vi "Device Params From Config XML File.vi"(8 "error IN":errorcluster, 11 "Configuration in":refnum<class "Configuration.lvclass">) -> (0 "error OUT":errorcluster, 1 "Device Settings":T2, 2 "Device Connections":T1, 3 "Configuration out":refnum<class "Configuration.lvclass">)   [LabVIEW 2011]
uses:
  Controls/Device Settings.ctl
  Controls/Device Connections.ctl
  Modules/File/Configuration/Configuration.lvclass
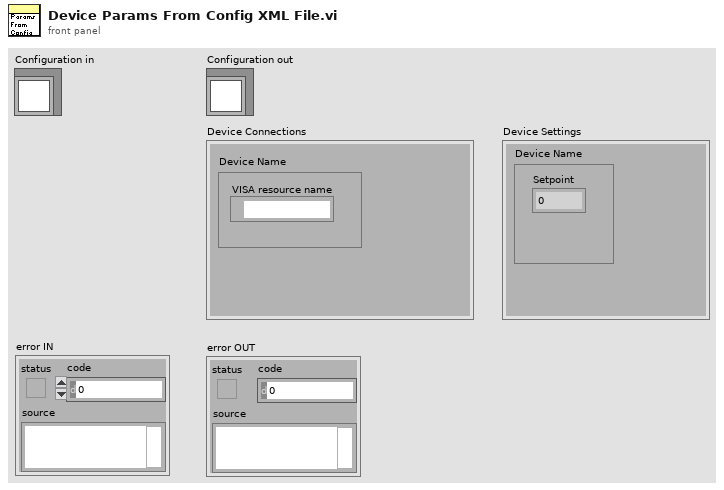
[diagram p1: front panel]
types:
  T1 = typedef "Device Connections.ctl" = cluster{"Device Name":cluster{"VISA resource name":refnum<visa-resource-name>}}
  T2 = typedef "Device Settings.ctl" = cluster{"Device Name":cluster{"Setpoint":dbl}}
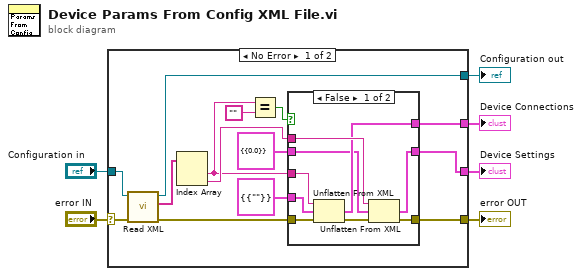
[diagram p0: block diagram]
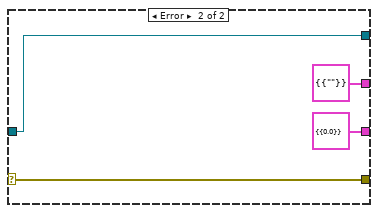
[diagram p3: hidden frame]
diagram:
  n1 = case shown="No Error" "error IN" {
    selector: "error IN" -> [w20 w35]
    tunnel: [w18 w36] -> w4
    tunnel: "Configuration in" -> [w19 w36]
    tunnel: [w15 w35] -> w5
    tunnel: [w14 T1 {"Device Name"={"VISA resource name"=""}} ("Device Connections")] -> w2
    tunnel: [w7 T2 {"Device Name"={"Setpoint"=0.0}} ("Device Settings")] -> w1
    frame No Error {
      n2 = call-dynamic "Read XML.vi"("error in (no error)"=w20, "Configuration in"=w19) -> ("error out"=w17:errorcluster, "XML Elements"=w12:string[], "Configuration out"=w18:refnum<class "Configuration.lvclass">)  [unwired: 7 in]
      n3 = Index Array(array=w12) -> (element #1=w10:string, element #2=w16:string)  [unwired: 2 in]
      n4 = Equal?(x=w10, y="") -> (x = y?=w11:bool)
      n5 = case shown="False" w11 {
        tunnel: w17 -> [w29 w30]
        tunnel: w16 -> [w27 _]
        tunnel: [w26 w30] -> w15
        tunnel: [w25 w32] -> w14
        tunnel: [w24 w31] -> w7
        tunnel: w10 -> [w23 _]
        tunnel: T1 {"Device Name"={"VISA resource name"=""}} ("Device Connections") -> [w22 w32]
        tunnel: T2 {"Device Name"={"Setpoint"=0.0}} ("Device Settings") -> [w21 w31]
        frame False {
          n6 = Unflatten From XML(xml string=w23, type=w22, error in (no error)=w29) -> (value=w25:T1, error out=w28:errorcluster)
          n7 = Unflatten From XML(xml string=w27, type=w21, error in (no error)=w28) -> (value=w24:T2, error out=w26:errorcluster)
        }
        frame True {
        }
      }
    }
    frame Error {
    }
  }
  "error OUT" <- w5
  "Device Settings" <- w1
  "Device Connections" <- w2
  "Configuration out" <- w4
